vi "Demo_CID_INDEX.vi"(1 "Index IN":i32) -> (0 "Index OUT":i32)   [LabVIEW 2017]
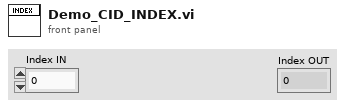
[diagram p1: front panel]
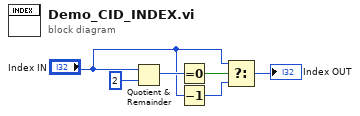
[diagram p0: block diagram]
diagram:
  n1 = Quotient & Remainder(x="Index IN", y=2) -> (x-y*floor(x/y)=w4:i32)  [unwired: 1 out]
  n2 = Equal To 0?(x=w4) -> (x = 0?=w5:bool)
  n3 = Decrement(x="Index IN") -> (x-1=w2:i32)
  n4 = Select(t="Index IN", s=w5, f=w2) -> (s? t:f=→"Index OUT":i32)
